vi "Is Micron sm130.vi"(8 "error in (no error)":errorcluster, 9 "Timeout":u32=10000, 10 "ID Query (True)":bool=TRUE, 11 "VISA resource name":refnum<visa-resource-name>) -> (0 "error out":errorcluster, 2 "Micron sm130":bool, 3 "VISA resource name out":refnum<visa-resource-name>)   [LabVIEW 2024]
doc: "Establishes communication with the instrument and optionally performs an instrument identification query and/or an instrument reset. It also places the instrument in a default state needed for other instrument driver operations. Therefore, call this VI before calling other instrument driver VIs for this instrument. Generally, you need to call the Initialize VI only once at the beginning of an application."
panel:
  # "(c) 2009 - 2012 National Instruments.  ALL RIGHTS RESERVED."
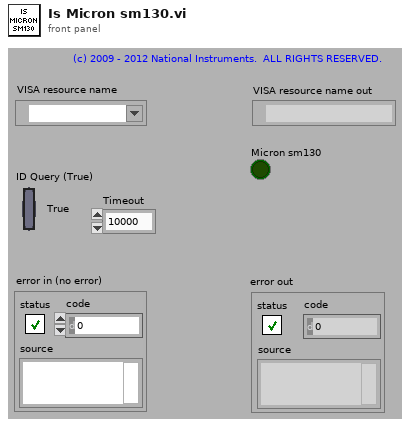
[diagram p1: front panel]
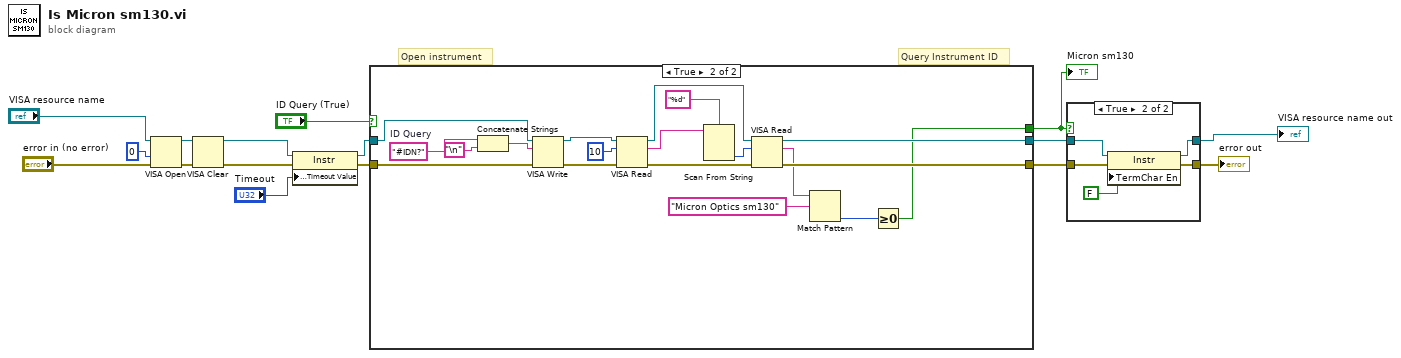
[diagram p0: block diagram]
diagram:
  # "Query Instrument ID"
  # "Open instrument"
  n1 = VISA Open(access mode=u32 0, error in (no error)="error in (no error)", VISA resource name="VISA resource name") -> (VISA resource name=w11:refnum<visa-resource-name>, error out=w10:errorcluster)  [unwired: 2 in]
  n2 = VISA Clear(VISA resource name=w11, error in (no error)=w10) -> (VISA resource name out=w9:refnum<visa-resource-name>, error out=w8:errorcluster)
  n3 = property class="Instr"(reference=w9, error in=w8, "General Settings:Timeout Value"="Timeout") -> (reference out=w7:refnum<visa-resource-name>, error out=w6:errorcluster)
  n4 = case shown="True" "ID Query (True)" {
    tunnel: [w17 w27] -> w5
    tunnel: [w18 w28] -> w3
    tunnel: w7 -> [w18 w36]
    tunnel: w6 -> [w17 w37]
    tunnel: [_ w19] -> w1
    frame False {
    }
    frame True {
      w22 = "#IDN?"  # ID Query
      n5 = Concatenate Strings(w22, "\n") -> (w20:string)
      n6 = VISA Write(VISA resource name=w36, write buffer=w20, error in (no error)=w37) -> (VISA resource name out=w35:refnum<visa-resource-name>, error out=w34:errorcluster)  [unwired: 1 out]
      n7 = VISA Read(VISA resource name=w35, byte count=u32 10, error in (no error)=w34) -> (VISA resource name out=w30:refnum<visa-resource-name>, read buffer=w26:string, error out=w29:errorcluster)  [unwired: 1 out]
      n8 = Scan From String(format string="%d", input string=w26) -> (output 1=w25:i32)  [unwired: 3 in, 3 out]
      n9 = VISA Read(VISA resource name=w30, byte count=w25, error in (no error)=w29) -> (VISA resource name out=w28:refnum<visa-resource-name>, read buffer=w23:string, error out=w27:errorcluster)  [unwired: 1 out]
      n10 = Match Pattern(string=w23, regular expression="Micron Optics sm130") -> (offset past match=w31:i32)  [unwired: 1 in, 3 out]
      n11 = Greater Or Equal To 0?(x=w31) -> (x >= 0?=w19:bool)
    }
  }
  "Micron sm130" <- w1
  n12 = case shown="True" w1 {
    tunnel: w5 -> [w38 w42]
    tunnel: [w38 w41] -> w4
    tunnel: w3 -> [w39 w44]
    tunnel: [w39 w43] -> w2
    frame False {
    }
    frame True {
      n13 = property class="Instr"(reference=w44, error in=w42, "TermChar En"=FALSE ("Message Based Settings:Termination Character Enable")) -> (reference out=w43:refnum<visa-resource-name>, error out=w41:errorcluster)
    }
  }
  "VISA resource name out" <- w2
  "error out" <- w4
